vi "Convert Real Time to Gate Time Option.vi"(2 "Lookup table":cluster{"Gate Time (us)":u32, "Gate Time":T1}[](array[cluster])=[{"Gate Time (us)"=50, "Gate Time"=2}, {"Gate Time (us)"=100, "Gate Time"=3}, {"Gate Time (us)"=200, "Gate Time"=4}, {"Gate Time (us)"=500, "Gate Time"=5}, {"Gate Time (us)"=1000, "Gate Time"=6}, {"Gate Time (us)"=2000, "Gate Time"=7}, {"Gate Time (us)"=5000, "Gate Time"=8}, {"Gate Time (us)"=10000, "Gate Time"=9}, {"Gate Time (us)"=20000, "Gate Time"=10}, {"Gate Time (us)"=50000, "Gate Time"=11}, {"Gate Time (us)"=100000, "Gate Time"=12}, {"Gate Time (us)"=200000, "Gate Time"=13}, {"Gate Time (us)"=500000, "Gate Time"=14}, {"Gate Time (us)"=1000000, "Gate Time"=15}, {"Gate Time (us)"=2000000, "Gate Time"=16}, {"Gate Time (us)"=5000000, "Gate Time"=17}, {"Gate Time (us)"=10000000, "Gate Time"=18}] {"Gate Time" items=["50u"=2, "100u"=3, "200u"=4, "500u"=5, "1m"=6, "2m"=7, "5m"=8, "10m"=9, "20m"=10, "50m"=11, "100m"=12, "200m"=13, "500m"=14, "1"=15, "2"=16, "5"=17, "10"=18]}, 3 "Gate Time (us)":u32) -> (1 "Gate Time":T1 items=["50u"=2, "100u"=3, "200u"=4, "500u"=5, "1m"=6, "2m"=7, "5m"=8, "10m"=9, "20m"=10, "50m"=11, "100m"=12, "200m"=13, "500m"=14, "1"=15, "2"=16, "5"=17, "10"=18])   [LabVIEW 2016, in "Drivers.lvlib" / "C8855-01.lvlib"]
uses:
  C8855-01.lvlib
  Gate Time.ctl
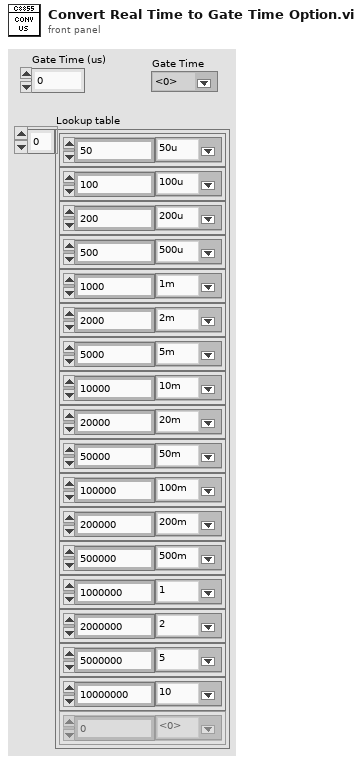
[diagram p1: front panel]
types:
  T1 = typedef "Drivers.lvlib/C8855-01.lvlib/Gate Time.ctl" = u8
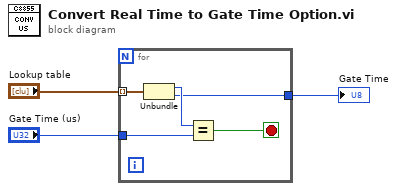
[diagram p0: block diagram]
diagram:
  n1 = for {
    tunnel: "Lookup table" -> [w8] mode=indexing
    tunnel: "Gate Time (us)" -> [w7]
    tunnel: [w5] -> w1
    stop <- w4 stop-if-true
    n2 = Unbundle(w8) -> ("Gate Time (us)"=w6:u32, "Gate Time"=w5:T1)
    n3 = Equal?(x=w6, y=w7) -> (x = y?=w4:bool)
  }
  "Gate Time" <- w1
